vi "SetAxisMotorType.vi"(8 "error in (no error)":errorcluster, 10 "MotorType":i32, 11 "Picomoto8742ControllerClass in":refnum<class "Picomoto8742ControllerClass.lvclass">) -> (0 "error out":errorcluster, 2 "Success?":bool, 3 "Picomoto8742ControllerClass out":refnum<class "Picomoto8742ControllerClass.lvclass">)   [LabVIEW 2013, in "Picomoto8742ControllerClass.lvclass"]
doc: "Send the motor type setting relative to the active axis, to the physical device"
uses:
  Picomoto8742ControllerClass.lvclass
  Picomoto8742ControllerClass.lvclass/Picomoto8742ControllerClass.ctl
  PicoMotor8742Axis/Picomotor8742Axis.lvclass
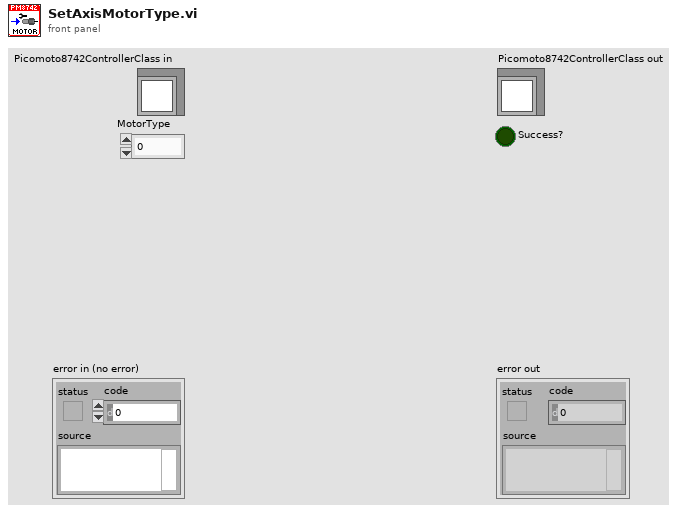
[diagram p1: front panel]
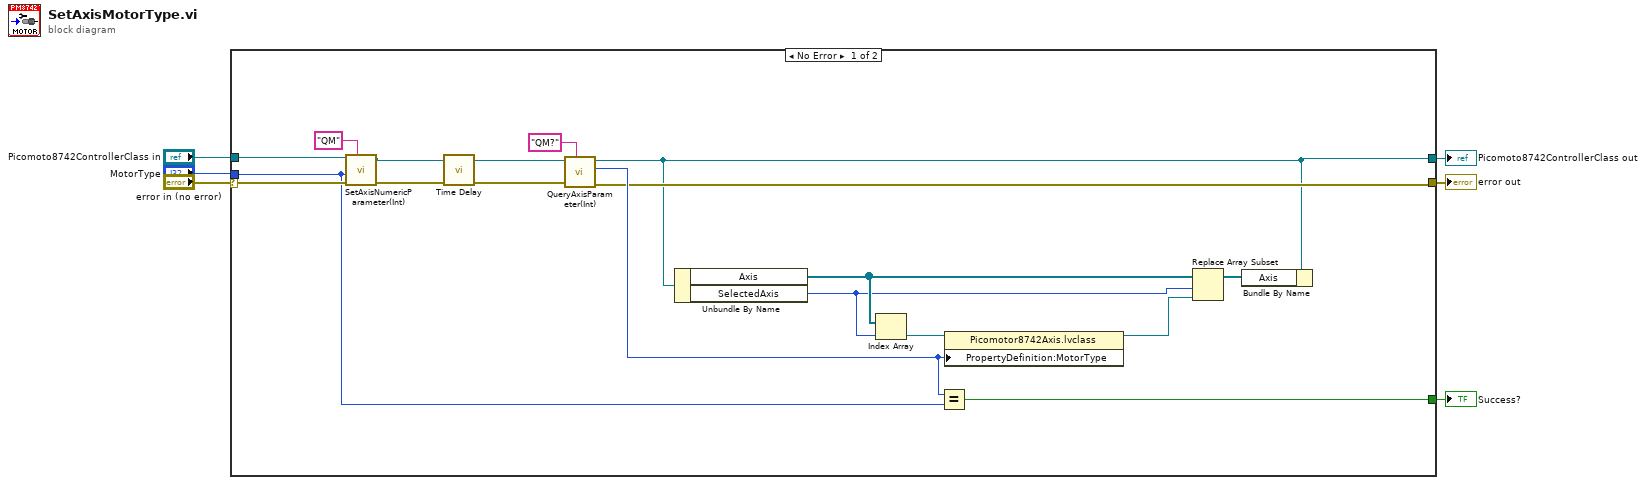
[diagram p0: block diagram]
diagram:
  n1 = case shown="No Error" "error in (no error)" {
    selector: "error in (no error)" -> [w23 w25]
    tunnel: [w8 w25] -> w5
    tunnel: [w7 w24] -> w3
    tunnel: "Picomoto8742ControllerClass in" -> [w22 w24]
    tunnel: "MotorType" -> [w10 _]
    tunnel: [w9 _] -> w1
    frame No Error {
      n2 = call "SetAxisNumericParameter(Int).vi"("CMD"="QM" ("string"), "error in (no error)"=w23, "ParameterValue"=w10, "Picomoto8742ControllerClass in"=w22) -> ("error out"=w20:errorcluster, "Picomoto8742ControllerClass Out"=w12:refnum<class "Picomoto8742ControllerClass.lvclass">)  [unwired: 6 in]
      n3 = call "Time Delay"("error in (no error)"=w20) -> ("error out"=w13:errorcluster)  [unwired: 10 in]
      n4 = call-dynamic "QueryAxisParameter(Int).vi"("Cmd"="QM?" ("string"), "error in (no error)"=w13, "Picomoto8742ControllerClass in"=w12) -> ("error out"=w8:errorcluster, "ValueOut"=w11:i32, "Picomoto8742ControllerClass Out"=w7:refnum<class "Picomoto8742ControllerClass.lvclass">)  [unwired: 6 in]
      n5 = Unbundle By Name(w7) -> ("Axis"=w16:refnum<class "Picomotor8742Axis.lvclass">[], "SelectedAxis"=w15:u32)
      n6 = Index Array(array=w16, index=w15) -> (element=w14:refnum<class "Picomotor8742Axis.lvclass">)
      n7 = Equal?(x=w11, y=w10) -> (x = y?=w9:bool)
      n8 = property class="Picomotor8742Axis.lvclass"(reference=w14, "PropertyDefinition:MotorType"=w11) -> (reference out=w19:refnum<class "Picomotor8742Axis.lvclass">)  [unwired: 1 in, 1 out]
      n9 = Replace Array Subset(array=w16, new element=w19, index=w15) -> (w18:refnum<class "Picomotor8742Axis.lvclass">[])
      n10 = Bundle By Name(cluster=w7, "Axis"=w18) -> ()  [unwired: 1 out]
    }
    frame Error {
    }
  }
  "error out" <- w5
  "Picomoto8742ControllerClass out" <- w3
  "Success?" <- w1
